vi "UpdateGraph.vi"(8 "error in (no error)":errorcluster caption="entrée d'erreur (pas d'erreur)", 10 "CurvesParams":T1[](array[typedef]), 11 "CurveIndexArr":i32[](array[numeric])) -> (0 "error out":errorcluster caption="sortie d'erreur", 2 "CurvesParamsOut":T1[](array[typedef]))   [LabVIEW 2010, in "Interface.lvclass"]
uses:
  Interface.lvclass
  CurveSetup.ctl
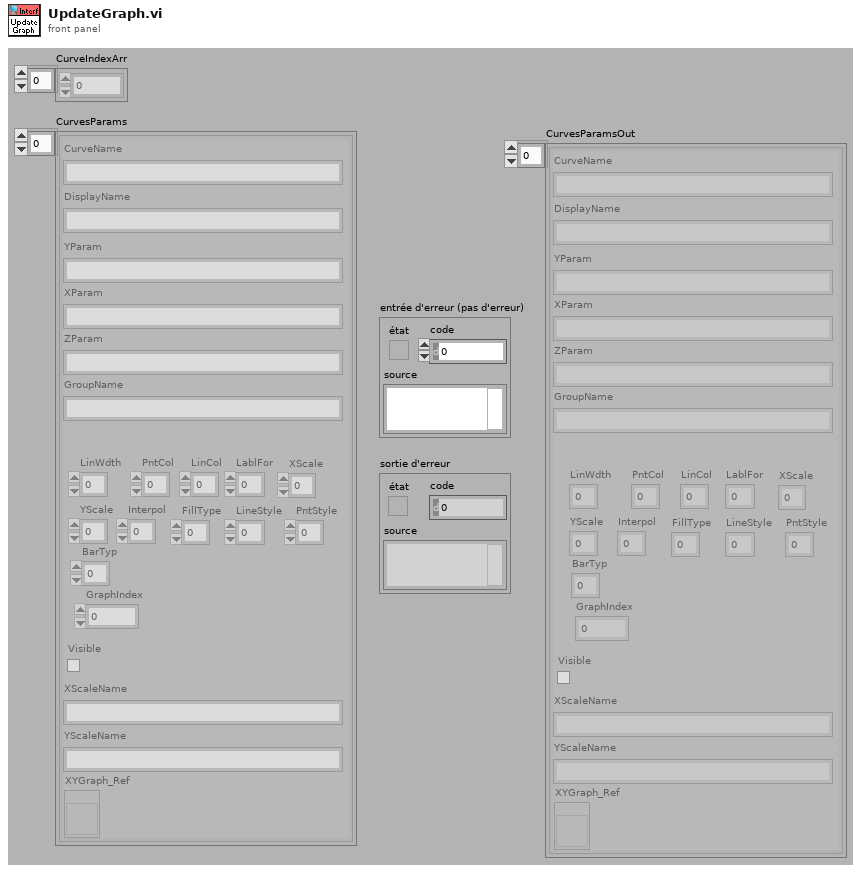
[diagram p1: front panel]
types:
  T1 = typedef "Interface.lvclass/CurveSetup.ctl" = cluster{"CurveName":string, "YParam":string, "XParam":string, "ZParam ":string, "GroupName":string, "LinWdth":u8, "PntCol":u32, "LinCol":u32, "LablFor":u8, "XScale":u32, "YScale":u32, "Interpol":u8, "DisplayName":string, "FillType":i16, "LineStyle":u8, "PntStyle":u8, "BarTyp":u8, "GraphIndex":i32, "Visible":bool, "XScaleName":string, "YScaleName":string, "XYGraph_Ref":refnum<vi>}
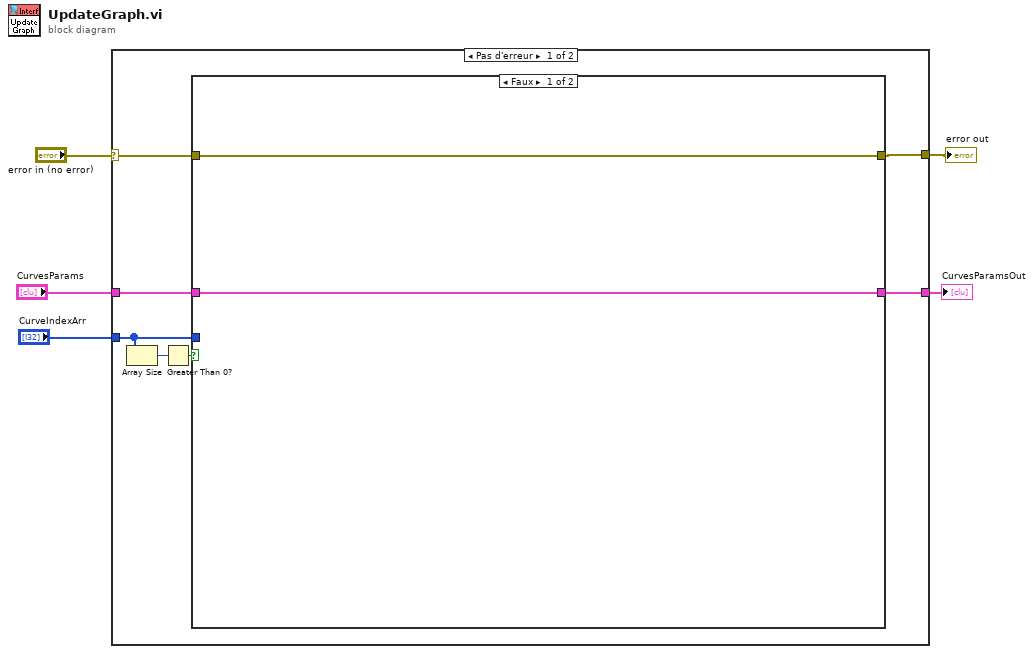
[diagram p0: block diagram]
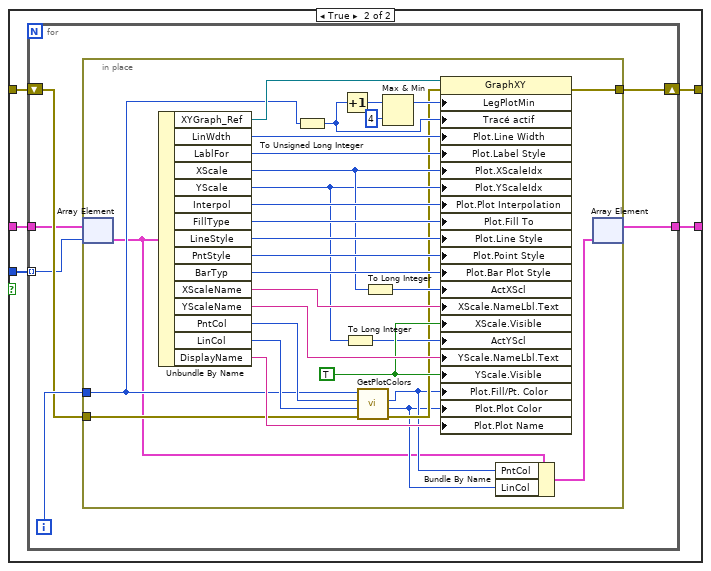
[diagram p2: hidden frame]
diagram:
  n1 = case shown="Pas d'erreur" "error in (no error)" {
    selector: "error in (no error)" -> [w10 w57]
    tunnel: [w12 w57] -> w4
    tunnel: "CurvesParams" -> [w11 w56]
    tunnel: "CurveIndexArr" -> [w8 _]
    tunnel: [w9 w56] -> w1
    frame No Error {
      n2 = Array Size(array=w8) -> (size(s)=w7:i32)
      n3 = Greater Than 0?(x=w7) -> (x > 0?=w6:bool)
      n4 = case shown="Faux" w6 {
        tunnel: [w13 w19] -> w12
        tunnel: w8 -> [_ w18]
        tunnel: w11 -> [w14 w17]
        tunnel: w10 -> [w13 w16]
        tunnel: [w14 w15] -> w9
        frame False {
        }
        frame True {
          n5 = for {
            tunnel: w17 -> [w23]
            tunnel: w18 -> [w22] mode=indexing
            shift-right: [w21] -> w19
            shift-left: w16 -> [w24]
            tunnel: [w20] -> w15
            i -> [w25]
            n6 = in-place {
              in-place-border: [w52] -> w21
              in-place-border: w25 -> [w32]
              in-place-border: w24 -> [w31]
              w51 = TRUE ("Échelle des Y.Visible")
              n7 = in-place-array #1(w23, w22) -> (w27:T1)
              n8 = Unbundle By Name(w27) -> ("XYGraph_Ref"=w35:refnum<vi>, "LinWdth"=w44:u8, "LablFor"=w45:u8, "XScale"=w43:u32, "YScale"=w41:u32, "Interpol"=w46:u8, "FillType"=w47:i16, "LineStyle"=w48:u8, "PntStyle"=w49:u8, "BarTyp"=w50:u8, "XScaleName"=w53:string, "YScaleName"=w54:string, "PntCol"=w34:u32, "LinCol"=w33:u32, "DisplayName"=w55:string)
              n9 = To Unsigned Long Integer(number=w32) -> (unsigned 32bit integer=w36:u32)
              n10 = Increment(x=w36) -> (x+1=w39:u32)
              n11 = To Long Integer(number=w41) -> (32bit integer=w40:i32)
              n12 = call "GetPlotColors.vi"("ErrorIn(No Error)"=w31, "Color2In"=w33, "Color1In"=w34, "ColorIndex"=w32) -> ("sortie d'erreur"=w30:errorcluster, "Color2Out"=w28:u32, "Color1Out"=w29:u32)  [unwired: 4 in, 1 out]
              n13 = To Long Integer(number=w43) -> (32bit integer=w42:i32)
              n14 = Max & Min(x=w39, y=u32 4) -> (max(x,y)=w37:u32)  [unwired: 1 out]
              n15 = property class="GraphXY"(reference=w35, error in=w30, "LegPlotMin"=w37, "Tracé actif"=w36, "Plot.Line Width"=w44, "Plot.Label Style"=w45, "Plot.XScaleIdx"=w43, "Plot.YScaleIdx"=w41, "Plot.Plot Interpolation"=w46, "Plot.Fill To"=w47, "Plot.Line Style"=w48, "Plot.Point Style"=w49, "Plot.Bar Plot Style"=w50, "ActXScl"=w42, "XScale.NameLbl.Text"=w53, "XScale.Visible"=w51, "ActYScl"=w40, "YScale.NameLbl.Text"=w54, "YScale.Visible"=w51, "Plot.Fill/Pt. Color"=w29, "Plot.Plot Color"=w28, "Plot.Plot Name"=w55) -> (error out=w52:errorcluster)  [unwired: 1 out]
              n16 = Bundle By Name(cluster=w27, "PntCol"=w29, "LinCol"=w28) -> (w26:T1)
              n17 = in-place-array #1(w26) -> (w20:T1[])  [unwired: 1 out]
            }
          }
        }
      }
    }
    frame Error {
    }
  }
  "error out" <- w4
  "CurvesParamsOut" <- w1
